vi "Result_Test.vi"(8 "error in (no error)":errorcluster caption="entrée d'erreur (pas d'erreur)", 11 "Flash_Jlink en entrée":refnum<class "Check_Temp.lvclass">) -> (0 "error out":errorcluster caption="sortie d'erreur", 3 "Flash_Jlink en sortie":refnum<class "Check_Temp.lvclass">)   [LabVIEW 2020, in "Library Test.lvlib" / "Check_Temp.lvclass"]
uses:
  Check_Temp.lvclass
  C:/Users/ngarcin/OneDrive - Altyor/Standard TB/Suite TB45/Class/Test/Test (Default)/Test (Default).lvclass
  Commun VI/TypeDef/Variable Printable.ctl
  Test_Without_Instr/Test_Without_Inst.lvclass
  Commun VI/Library Commun.lvlib
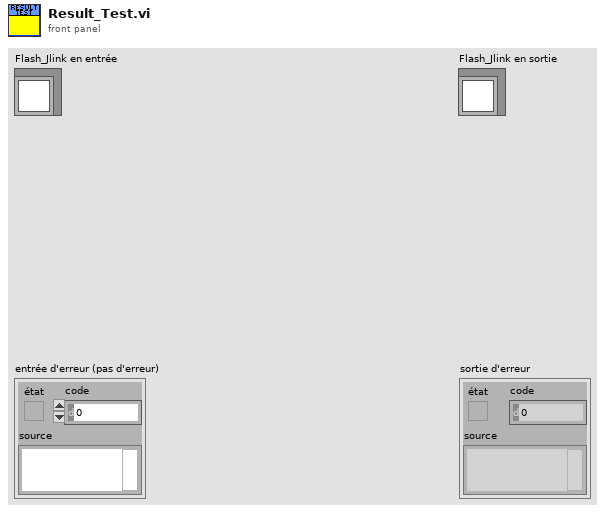
[diagram p1: front panel]
types:
  T1 = enum16{"Get Variable", "Get All Variables", "Set Variable", "Delete Variable", "Delete All Variable"}
  T2 = typedef "Variable Printable.ctl" = string
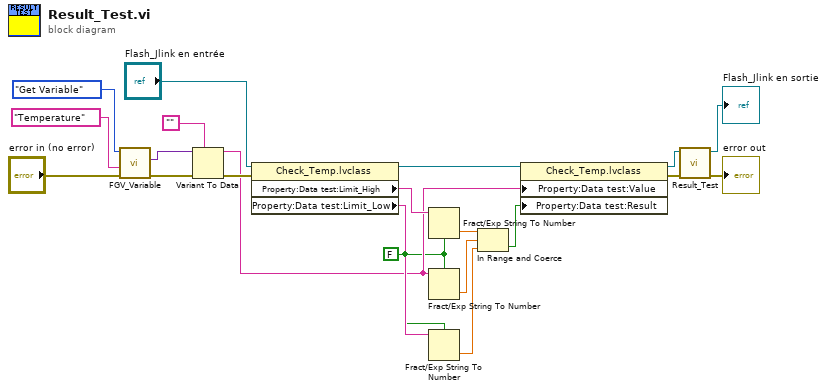
[diagram p0: block diagram]
diagram:
  w5 = FALSE ("utiliser le séparateur décimal du système (V)")
  n1 = call "FGV_Variable.vi"("error in (no error)"="error in (no error)", "Variable"=T2 "Temperature", "Function"=T1."Get Variable") -> ("error out"=w14:errorcluster, "Data Out"=w13:variant)  [unwired: 6 in, 1 out]
  n2 = Variant To Data(error in=w14, type="", Variant=w13) -> (data=w6:string, error out=w11:errorcluster)
  n3 = property class="Check_Temp.lvclass"(reference="Flash_Jlink en entrée", error in=w11) -> (reference out=w10:refnum<class "Check_Temp.lvclass">, "Property:Data test:Limit_High"=w8:string, "Property:Data test:Limit_Low"=w7:string)  [unwired: 1 out]
  n4 = Fract/Exp String To Number(use system decimal point (T)=w5, string=w8) -> (number=w4:dbl)  [unwired: 2 in, 1 out]
  n5 = Fract/Exp String To Number(use system decimal point (T)=w5, string=w6) -> (number=w2:dbl)  [unwired: 2 in, 1 out]
  n6 = Fract/Exp String To Number(use system decimal point (T)=w5, string=w7) -> (number=w3:dbl)  [unwired: 2 in, 1 out]
  n7 = In Range and Coerce(upper limit=w4, x=w2, lower limit=w3) -> (In Range?=w1:bool)  [unwired: 1 out]
  n8 = property class="Check_Temp.lvclass"(reference=w10, "Property:Data test:Value"=w6, "Property:Data test:Result"=w1) -> (reference out=w18:refnum<class "Check_Temp.lvclass">, error out=w19:errorcluster)  [unwired: 1 in]
  n9 = call-parent "Result_Test.vi"("error in (no error)"=w19, "Test_Without_Inst en entrée"=w18) -> ("error out"=→"error out":errorcluster, "Test_Without_Inst en sortie"=→"Flash_Jlink en sortie":refnum<class "Check_Temp.lvclass">)  [unwired: 8 in]
